vi "Read_data.vi"() -> ()   [LabVIEW 2020]
panel:
  out "Signals":dynamicdata(graph)
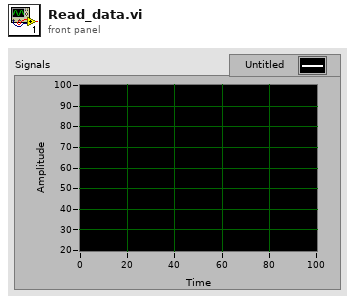
[diagram p1: front panel]
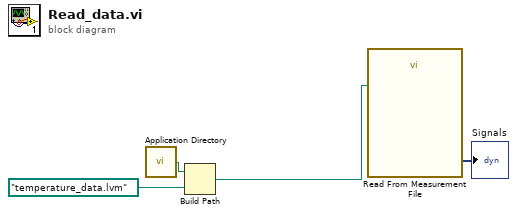
[diagram p0: block diagram]
diagram:
  n1 = call <vilib>:"Application Directory.vi"() -> ("Application Directory"=w3:path)
  n2 = Build Path(base path=w3, name or relative path=path "temperature_data.lvm") -> (appended path=w2:path)
  n3 = call "Read From Measurement File"("Filename"=w2) -> ("Signals"=→"Signals":dynamicdata)  [unwired: 5 in, 5 out]
